vi "Get Item Test.vi"() -> ()   [LabVIEW 2017]
uses:
  String Subset.vi
  Parsing/Parse Full Path or Item Name.vi
  Offset/Find Item Locations by Path.vi
  <vilib>/addons/_JKI Toolkits/Caraya/classes/Assert/Assert.lvclass
  <vilib>/addons/_JKI Toolkits/Caraya/classes/Test/Test.lvclass
  JSONtext.lvlib
panel:
  out "Array 2":string[](array[string])
  out "Array":bool[](array[boolean])
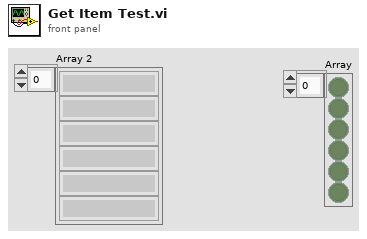
[diagram p1: front panel]
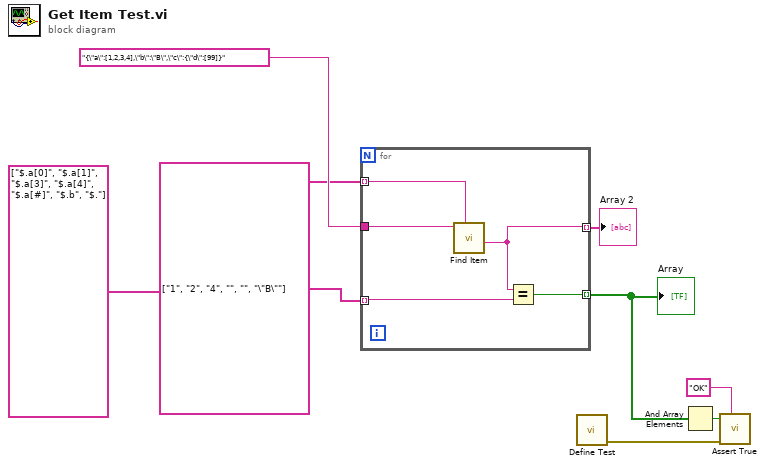
[diagram p0: block diagram]
diagram:
  n1 = for {
    tunnel: "{\"a\":[1,2,3,4],\"b\":\"B\",\"c\":{\"d\":[99]}" -> [w10]
    tunnel: string[] ["$.a[0]", "$.a[1]", "$.a[3]", "$.a[4]", "$.a[#]", "$.b", "$."] -> [w11] mode=indexing
    tunnel: string[] ["1", "2", "4", "", "", "\"B\""] -> [w13] mode=indexing
    tunnel: [w12] -> w1 mode=indexing
    tunnel: [w9] -> w5 mode=indexing
    n2 = call "Find Item.vi"("$Path or Item Name"=w11, "JSON"=w10) -> ("<JSON>"=w9:string)  [unwired: 6 in, 3 out]
    n3 = Equal?(x=w9, y=w13) -> (x = y?=w12:bool)
  }
  "Array" <- w1
  "Array 2" <- w5
  n4 = call <vilib>:"Define Test.vi"() -> ("error out"=w2:errorcluster)  [unwired: 11 in]
  n5 = And Array Elements(Boolean array=w1) -> (logical AND=w4:bool)
  n6 = call <vilib>:"Assert True.vi"("Label"="OK", "error in (no error)"=w2, "True?"=w4) -> ()  [unwired: 8 in, 1 out]
